vi "Unmarshal.vi"(8 "error in (no error)":errorcluster, 10 "Buffer":u8[](array[numeric]), 11 "int32 in":refnum<class "float.lvclass">) -> (0 "error out":errorcluster, 2 "Buffer Count":i32=4, 3 "int32 out":refnum<class "float.lvclass">)   [LabVIEW 2020, in "Protobuf RAW.lvlib" / "float.lvclass"]
uses:
  float.lvclass
  float.lvclass/float.ctl
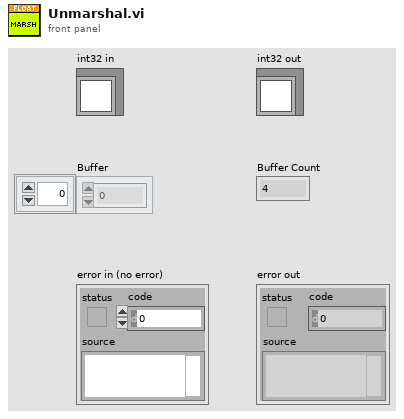
[diagram p1: front panel]
types:
  T1 = enum16{"big-endian, network order", "native, host order", "little-endian"}
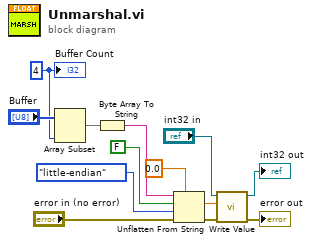
[diagram p0: block diagram]
diagram:
  w8 = 4 ("Buffer Count")
  n1 = Array Subset(array="Buffer", length=w8) -> (w9:u8[])  [unwired: 1 in]
  n2 = Byte Array To String(unsigned byte array=w9) -> (string=w5:string)
  n3 = Unflatten From String(type=sgl 0.0 ("Value"), binary string=w5, data includes array or string size? (T)=FALSE, byte order (0:big-endian, network order)=T1."little-endian", error in (no error)="error in (no error)") -> (value=w1:sgl, error out=w11:errorcluster)  [unwired: 1 out]
  n4 = call "Write Value.vi"("error in (no error)"=w11, "Value"=w1, "float in"="int32 in") -> ("error out"=→"error out":errorcluster, "float out"=→"int32 out":refnum<class "float.lvclass">)  [unwired: 7 in]
  "Buffer Count" <- w8
